vi "Format CSV.vi"(8 "error in (no error)":errorcluster, 9 "delimiter":string=",", 10 "CSV File Input":path, 11 "Original CSV Format":enum16{"Format A", "Format B"}(ring)) -> (0 "error out":errorcluster, 1 "Parcel Length":i32[](array[numeric]), 2 "All Terminal Data":T1(array[cluster]))   [LabVIEW 2017] (continued)
"36:44.6", "36:44.6", "36:44.6", "36:44.7", "36:44.7", "36:44.7", "36:44.8", "36:44.8", "36:44.8", "36:44.9", "36:44.9", "36:44.9", "36:45.0", "36:45.0", "36:45.0", "36:45.1", "36:45.1", "36:45.1", "36:45.2", "36:45.2", "36:45.2", "36:45.3", "36:45.3", "36:45.3", "36:45.4", "36:45.4", "36:45.4", "36:45.5", "36:45.5", "36:45.5", "36:45.6", "36:45.6", "36:45.6", "36:45.7", "36:45.7", "36:45.7", "36:45.8", "36:45.8", "36:45.8", "36:45.9", "36:45.9", "36:45.9", "36:46.0", "36:46.0", "36:46.0", "36:46.1", "36:46.1", "36:46.1", "36:46.2", "36:46.2", "36:46.2", "36:46.3", "36:46.3", "36:46.3", "36:46.4", "36:46.4", "36:46.4", "36:46.5", "36:46.5", "36:46.5", "36:46.6", "36:46.6", "36:46.6", "36:46.7", "36:46.7", "36:46.7", "36:46.8", "36:46.8", "36:46.8", "36:46.9", "36:46.9", "36:46.9", "36:47.0", "36:47.0", "36:47.0", "36:47.1", "36:47.1", "36:47.1", "36:47.2", "36:47.2", "36:47.2", "36:47.3", "36:47.3", "36:47.3", "36:47.4", "36:47.4", "36:47.4", "36:47.5", "36:47.5", "36:47.5", "36:47.6", "36:47.6", "36:47.6", "36:47.7", "36:47.7", "36:47.7", "36:47.8", "36:47.8", "36:47.8", "36:47.9", "36:47.9", "36:47.9", "36:48.0", "36:48.0", "36:48.0", "36:48.1", "36:48.1", "36:48.1", "36:48.2", "36:48.2", "36:48.2", "36:48.3", "36:48.3", "36:48.3", "36:48.4", "36:48.4", "36:48.4", "36:48.5", "36:48.5", "36:48.5", "36:48.6", "36:48.6", "36:48.6", "36:48.7", "36:48.7", "36:48.7", "36:48.8", "36:48.8", "36:48.8", "36:48.9", "36:48.9", "36:48.9", "36:49.0", "36:49.0", "36:49.0", "36:49.1", "36:49.1", "36:49.1", "36:49.2", "36:49.2", "36:49.2", "36:49.3", "36:49.3", "36:49.3", "36:49.4", "36:49.4", "36:49.4", "36:49.5", "36:49.5", "36:49.5", "36:49.6", "36:49.6", "36:49.6", "36:49.7", "36:49.7", "36:49.7", "36:49.8", "36:49.8", "36:49.8", "36:49.9", "36:49.9", "36:49.9", "36:50.0", "36:50.0", "36:50.0", "36:50.1", "36:50.1", "36:50.1", "36:50.2", "36:50.2", "36:50.2", "36:50.3", "36:50.3", "36:50.3", "36:50.4", "36:50.4", "36:50.4", "36:50.5", "36:50.5", "36:50.5", "36:50.6", "36:50.6", "36:50.6", "36:50.7", "36:50.7", "36:50.7", "36:50.8", "36:50.8", "36:50.8", "36:50.9", "36:50.9", "36:50.9", "36:51.0", "36:51.0", "36:51.0", "36:51.1", "36:51.1", "36:51.1", "36:51.2", "36:51.2", "36:51.2", "36:51.3", "36:51.3", "36:51.3", "36:51.4", "36:51.4", "36:51.4", "36:51.5", "36:51.5", "36:51.5", "36:51.6", "36:51.6", "36:51.6", "36:51.7", "36:51.7", "36:51.7", "36:51.8", "36:51.8", "36:51.8", "36:51.9", "36:51.9", "36:51.9", "36:52.0", "36:52.0", "36:52.0", "36:52.1", "36:52.1", "36:52.1", "36:52.2", "36:52.2", "36:52.2", "36:52.3", "36:52.3", "36:52.3", "36:52.4", "36:52.4", "36:52.4", "36:52.5", "36:52.5", "36:52.5", "36:52.6", "36:52.6", "36:52.6", "36:52.7", "36:52.7", "36:52.7", "36:52.8", "36:52.8", "36:52.8", "36:52.9", "36:52.9", "36:52.9", "36:53.0", "36:53.0", "36:53.0", "36:53.1", "36:53.1", "36:53.1", "36:53.2", "36:53.2", "36:53.2", "36:53.3", "36:53.3", "36:53.3", "36:53.4", "36:53.4", "36:53.4", "36:53.5", "36:53.5", "36:53.5", "36:53.6", "36:53.6", "36:53.6", "36:53.7", "36:53.7", "36:53.7", "36:53.8", "36:53.8", "36:53.8", "36:53.9", "36:53.9", "36:53.9", "36:54.0", "36:54.0", "36:54.0", "36:54.1", "36:54.1", "36:54.1", "36:54.2", "36:54.2", "36:54.2", "36:54.3", "36:54.3", "36:54.3", "36:54.4", "36:54.4", "36:54.4", "36:54.5", "36:54.5", "36:54.5", "36:54.6", "36:54.6", "36:54.6", "36:54.7", "36:54.7", "36:54.7", "36:54.8", "36:54.8", "36:54.8", "36:54.9", "36:54.9", "36:54.9", "36:55.0", "36:55.0", "36:55.0", "36:55.1", "36:55.1", "36:55.1", "36:55.2", "36:55.2", "36:55.2", "36:55.3", "36:55.3", "36:55.3", "36:55.4", "36:55.4", "36:55.4", "36:55.5", "36:55.5", "36:55.5", "36:55.6", "36:55.6", "36:55.6", "36:55.7", "36:55.7", "36:55.7", "36:55.8", "36:55.8", "36:55.8", "36:55.9", "36:55.9", "36:55.9", "36:56.0", "36:56.0", "36:56.0", "36:56.1", "36:56.1", "36:56.1", "36:56.2", "36:56.2", "36:56.2", "36:56.3", "36:56.3", "36:56.3", "36:56.4", "36:56.4", "36:56.4", "36:56.5", "36:56.5", "36:56.5", "36:56.6", "36:56.6", "36:56.6", "36:56.7", "36:56.7", "36:56.7", "36:56.8", "36:56.8", "36:56.8", "36:56.9", "36:56.9", "36:56.9", "36:57.0", "36:57.0", "36:57.0", "36:57.1", "36:57.1", "36:57.1", "36:57.2", "36:57.2", "36:57.2", "36:57.3", "36:57.3", "36:57.3", "36:57.4", "36:57.4", "36:57.4", "36:57.5", "36:57.5", "36:57.5", "36:57.6", "36:57.6", "36:57.6", "36:57.7", "36:57.7", "36:57.7", "36:57.8", "36:57.8", "36:57.8", "36:57.9", "36:57.9", "36:57.9", "36:58.0", "36:58.0", "36:58.0", "36:58.1", "36:58.1", "36:58.1", "36:58.2", "36:58.2", "36:58.2", "36:58.3", "36:58.3", "36:58.3", "36:58.4", "36:58.4", "36:58.4", "36:58.5", "36:58.5", "36:58.5", "36:58.6", "36:58.6", "36:58.6", "36:58.7", "36:58.7", "36:58.7", "36:58.8", "36:58.8", "36:58.8", "36:58.9", "36:58.9", "36:58.9", "36:59.0", "36:59.0", "36:59.0", "36:59.1", "36:59.1", "36:59.1", "36:59.2", "36:59.2", "36:59.2", "36:59.3", "36:59.3", "36:59.3", "36:59.4", "36:59.4", "36:59.4", "36:59.5", "36:59.5", "36:59.5", "36:59.6", "36:59.6", "36:59.6", "36:59.7", "36:59.7", "36:59.7", "36:59.8", "36:59.8", "36:59.8", "36:59.9", "36:59.9", "36:59.9", "37:00.0", "37:00.0", "37:00.0", "37:00.1", "37:00.1", "37:00.1", "37:00.2", "37:00.2", "37:00.2", "37:00.3", "37:00.3", "37:00.3", "37:00.4", "37:00.4", "37:00.4", "37:00.5", "37:00.5", "37:00.5", "37:00.6", "37:00.6", "37:00.6", "37:00.7", "37:00.7", "37:00.7", "37:00.8", "37:00.8", "37:00.8", "37:00.9", "37:00.9", "37:00.9", "37:01.0", "37:01.0", "37:01.0", "37:01.1", "37:01.1", "37:01.1", "37:01.2", "37:01.2", "37:01.2", "37:01.3", "37:01.3", "37:01.3", "37:01.4", "37:01.4", "37:01.4", "37:01.5", "37:01.5", "37:01.5", "37:01.6", "37:01.6", "37:01.6", "37:01.7", "37:01.7", "37:01.7", "37:01.8", "37:01.8", "37:01.8", "37:01.9", "37:01.9", "37:01.9", "37:02.0", "37:02.0", "37:02.0", "37:02.1", "37:02.1", "37:02.1", "37:02.2", "37:02.2", "37:02.2", "37:02.3", "37:02.3", "37:02.3", "37:02.4", "37:02.4", "37:02.4", "37:02.5", "37:02.5", "37:02.5", "37:02.6", "37:02.6", "37:02.6", "37:02.7", "37:02.7", "37:02.7", "37:02.8", "37:02.8", "37:02.8", "37:02.9", "37:02.9", "37:02.9", "37:03.0", "37:03.0", "37:03.0", "37:03.1", "37:03.1", "37:03.1", "37:03.2", "37:03.2", "37:03.2", "37:03.3", "37:03.3", "37:03.3", "37:03.4", "37:03.4", "37:03.4", "37:03.5", "37:03.5", "37:03.5", "37:03.6", "37:03.6", "37:03.6", "37:03.7", "37:03.7", "37:03.7", "37:03.8", "37:03.8", "37:03.8", "37:03.9", "37:03.9", "37:03.9", "37:04.0", "37:04.0", "37:04.0", "37:04.1", "37:04.1", "37:04.1", "37:04.2", "37:04.2", "37:04.2", "37:04.3", "37:04.3", "37:04.3", "37:04.4", "37:04.4", "37:04.4", "37:04.5", "37:04.5", "37:04.5", "37:04.6", "37:04.6", "37:04.6", "37:04.7", "37:04.7", "37:04.7", "37:04.8", "37:04.8", "37:04.8", "37:04.9", "37:04.9", "37:04.9", "37:05.0", "37:05.0", "37:05.0", "37:05.1", "37:05.1", "37:05.1", "37:05.2", "37:05.2", "37:05.2", "37:05.3", "37:05.3", "37:05.3", "37:05.4", "37:05.4", "37:05.4", "37:05.5", "37:05.5", "37:05.5", "37:05.6", "37:05.6", "37:05.6", "37:05.7", "37:05.7", "37:05.7", "37:05.8", "37:05.8", "37:05.8", "37:05.9", "37:05.9", "37:05.9", "37:06.0", "37:06.0", "37:06.0", "37:06.1", "37:06.1", "37:06.1", "37:06.2", "37:06.2", "37:06.2", "37:06.3", "37:06.3", "37:06.3", "37:06.4", "37:06.4", "37:06.4", "37:06.5", "37:06.5", "37:06.5", "37:06.6", "37:06.6", "37:06.6", "37:06.7", "37:06.7", "37:06.7", "37:06.8", "37:06.8", "37:06.8", "37:06.9", "37:06.9", "37:06.9", "37:07.0", "37:07.0", "37:07.0", "37:07.1", "37:07.1", "37:07.1", "37:07.2", "37:07.2", "37:07.2", "37:07.3", "37:07.3", "37:07.3", "37:07.4", "37:07.4", "37:07.4", "37:07.5", "37:07.5", "37:07.5", "37:07.6", "37:07.6", "37:07.6", "37:07.7", "37:07.7", "37:07.7", "37:07.8", "37:07.8", "37:07.8", "37:07.9", "37:07.9", "37:07.9", "37:08.0", "37:08.0", "37:08.0", "37:08.1", "37:08.1", "37:08.1", "37:08.2", "37:08.2", "37:08.2", "37:08.3", "37:08.3", "37:08.3", "37:08.4", "37:08.4", "37:08.4", "37:08.5", "37:08.5", "37:08.5", "37:08.6", "37:08.6", "37:08.6", "37:08.7", "37:08.7", "37:08.7", "37:08.8", "37:08.8", "37:08.8", "37:08.9", "37:08.9", "37:08.9", "37:09.0", "37:09.0", "37:09.0", "37:09.1", "37:09.1", "37:09.1", "37:09.2", "37:09.2", "37:09.2", "37:09.3", "37:09.3", "37:09.3", "37:09.4", "37:09.4", "37:09.4", "37:09.5", "37:09.5", "37:09.5", "37:09.6", "37:09.6", "37:09.6", "37:09.7", "37:09.7", "37:09.7", "37:09.8", "37:09.8", "37:09.8", "37:09.9", "37:09.9", "37:09.9", "37:10.0", "37:10.0", "37:10.0", "37:10.1", "37:10.1", "37:10.1", "37:10.2", "37:10.2", "37:10.2", "37:10.3", "37:10.3", "37:10.3", "37:10.4", "37:10.4", "37:10.4", "37:10.5", "37:10.5", "37:10.5", "37:10.6", "37:10.6", "37:10.6", "37:10.7", "37:10.7", "37:10.7", "37:10.8", "37:10.8", "37:10.8", "37:10.9", "37:10.9", "37:10.9", "37:11.0", "37:11.0", "37:11.0", "37:11.1", "37:11.1", "37:11.1", "37:11.2", "37:11.2", "37:11.2", "37:11.3", "37:11.3", "37:11.3", "37:11.4", "37:11.4", "37:11.4", "37:11.5", "37:11.5", "37:11.5", "37:11.6", "37:11.6", "37:11.6", "37:11.7", "37:11.7", "37:11.7", "37:11.8", "37:11.8", "37:11.8", "37:11.9", "37:11.9", "37:11.9", "37:12.0", "37:12.0", "37:12.0", "37:12.1", "37:12.1", "37:12.1", "37:12.2", "37:12.2", "37:12.2", "37:12.3", "37:12.3", "37:12.3", "37:12.4", "37:12.4", "37:12.4", "37:12.5", "37:12.5", "37:12.5", "37:12.6", "37:12.6", "37:12.6", "37:12.7", "37:12.7", "37:12.7", "37:12.8", "37:12.8", "37:12.8", "37:12.9", "37:12.9", "37:12.9", "37:13.0", "37:13.0", "37:13.0", "37:13.1", "37:13.1", "37:13.1", "37:13.2", "37:13.2", "37:13.2", "37:13.3", "37:13.3", "37:13.3", "37:13.4", "37:13.4", "37:13.4", "37:13.5", "37:13.5", "37:13.5", "37:13.6", "37:13.6", "37:13.6", "37:13.7", "37:13.7", "37:13.7", "37:13.8", "37:13.8", "37:13.8", "37:13.9", "37:13.9", "37:13.9", "37:14.0", "37:14.0", "37:14.0", "37:14.1", "37:14.1", "37:14.1", "37:14.2", "37:14.2", "37:14.2", "37:14.3", "37:14.3", "37:14.3", "37:14.4", "37:14.4", "37:14.4", "37:14.5", "37:14.5", "37:14.5", "37:14.6", "37:14.6", "37:14.6", "37:14.7", "37:14.7", "37:14.7", "37:14.8", "37:14.8", "37:14.8", "37:14.9", "37:14.9", "37:14.9", "37:15.0", "37:15.0", "37:15.0", "37:15.1", "37:15.1", "37:15.1", "37:15.2", "37:15.2", "37:15.2", "37:15.3", "37:15.3", "37:15.3", "37:15.4", "37:15.4", "37:15.4", "37:15.5", "37:15.5", "37:15.5", "37:15.6", "37:15.6", "37:15.6", "37:15.7", "37:15.7", "37:15.7", "37:15.8", "37:15.8", "37:15.8", "37:15.9", "37:15.9", "37:15.9", "37:16.0", "37:16.0", "37:16.0", "37:16.1", "37:16.1", "37:16.1", "37:16.2", "37:16.2", "37:16.2", "37:16.3", "37:16.3", "37:16.3", "37:16.4", "37:16.4", "37:16.4", "37:16.5", "37:16.5", "37:16.5", "37:16.6", "37:16.6", "37:16.6", "37:16.7", "37:16.7", "37:16.7", "37:16.8", "37:16.8", "37:16.8", "37:16.9", "37:16.9", "37:16.9", "37:17.0", "37:17.0", "37:17.0", "37:17.1", "37:17.1", "37:17.1", "37:17.2", "37:17.2", "37:17.2", "37:17.3", "37:17.3", "37:17.3", "37:17.4", "37:17.4", "37:17.4", "37:17.5", "37:17.5", "37:17.5", "37:17.6", "37:17.6", "37:17.6", "37:17.7", "37:17.7", "37:17.7", "37:17.8", "37:17.8", "37:17.8", "37:17.9", "37:17.9", "37:17.9", "37:18.0", "37:18.0", "37:18.0", "37:18.1", "37:18.1", "37:18.1", "37:18.2", "37:18.2", "37:18.2", "37:18.3", "37:18.3", "37:18.3", "37:18.4", "37:18.4", "37:18.4", "37:18.5", "37:18.5", "37:18.5", "37:18.6", "37:18.6", "37:18.6", "37:18.7", "37:18.7", "37:18.7", "37:18.8", "37:18.8", "37:18.8", "37:18.9", "37:18.9", "37:18.9", "37:19.0", "37:19.0", "37:19.0", "37:19.1", "37:19.1", "37:19.1", "37:19.2", "37:19.2", "37:19.2", "37:19.3", "37:19.3", "37:19.3", "37:19.4", "37:19.4", "37:19.4", "37:19.5", "37:19.5", "37:19.5", "37:19.6", "37:19.6", "37:19.6", "37:19.7", "37:19.7", "37:19.7", "37:19.8", "37:19.8", "37:19.8", "37:19.9", "37:19.9", "37:19.9", "37:20.0", "37:20.0", "37:20.0", "37:20.1", "37:20.1", "37:20.1", "37:20.2", "37:20.2", "37:20.2", "37:20.3", "37:20.3", "37:20.3", "37:20.4", "37:20.4", "37:20.4", "37:20.5", "37:20.5", "37:20.5", "37:20.6", "37:20.6", "37:20.6", "37:20.7", "37:20.7", "37:20.7", "37:20.8", "37:20.8", "37:20.8", "37:20.9", "37:20.9", "37:20.9", "37:21.0", "37:21.0", "37:21.0", "37:21.1", "37:21.1", "37:21.1", "37:21.2", "37:21.2", "37:21.2", "37:21.3", "37:21.3", "37:21.3", "37:21.4", "37:21.4", "37:21.4", "37:21.5", "37:21.5", "37:21.5", "37:21.6", "37:21.6", "37:21.6", "37:21.7", "37:21.7", "37:21.7", "37:21.8", "37:21.8", "37:21.8", "37:21.9", "37:21.9", "37:21.9", "37:22.0", "37:22.0", "37:22.0", "37:22.1", "37:22.1", "37:22.1", "37:22.2", "37:22.2", "37:22.2", "37:22.3", "37:22.3", "37:22.3", "37:22.4", "37:22.4", "37:22.4", "37:22.5", "37:22.5", "37:22.5", "37:22.6", "37:22.6", "37:22.6", "37:22.7", "37:22.7", "37:22.7", "37:22.8", "37:22.8", "37:22.8", "37:22.9", "37:22.9", "37:22.9", "37:23.0", "37:23.0", "37:23.0", "37:23.1", "37:23.1", "37:23.1", "37:23.2", "37:23.2", "37:23.2", "37:23.3", "37:23.3", "37:23.3", "37:23.4", "37:23.4", "37:23.4", "37:23.5", "37:23.5", "37:23.5", "37:23.6", "37:23.6", "37:23.6", "37:23.7", "37:23.7", "37:23.7", "37:23.8", "37:23.8", "37:23.8", "37:23.9", "37:23.9", "37:23.9", "37:24.0", "37:24.0", "37:24.0", "37:24.1", "37:24.1", "37:24.1", "37:24.2", "37:24.2", "37:24.2", "37:24.3", "37:24.3", "37:24.3", "37:24.4", "37:24.4", "37:24.4", "37:24.5", "37:24.5", "37:24.5", "37:24.6", "37:24.6", "37:24.6", "37:24.7", "37:24.7", "37:24.7", "37:24.8", "37:24.8", "37:24.8", "37:24.9", "37:24.9", "37:24.9", "37:25.0", "37:25.0", "37:25.0", "37:25.1", "37:25.1", "37:25.1", "37:25.2", "37:25.2", "37:25.2", "37:25.3", "37:25.3", "37:25.3", "37:25.4", "37:25.4", "37:25.4", "37:25.5", "37:25.5", "37:25.5", "37:25.6", "37:25.6", "37:25.6", "37:25.7", "37:25.7", "37:25.7", "37:25.8", "37:25.8", "37:25.8", "37:25.9", "37:25.9", "37:25.9", "37:26.0", "37:26.0", "37:26.0", "37:26.1", "37:26.1", "37:26.1", "37:26.2", "37:26.2", "37:26.2", "37:26.3", "37:26.3", "37:26.3", "37:26.4", "37:26.4", "37:26.4", "37:26.5", "37:26.5", "37:26.5", "37:26.6", "37:26.6", "37:26.6", "37:26.7", "37:26.7", "37:26.7", "37:26.8", "37:26.8", "37:26.8", "37:26.9", "37:26.9", "37:26.9", "37:27.0", "37:27.0", "37:27.0", "37:27.1", "37:27.1", "37:27.1", "37:27.2", "37:27.2", "37:27.2", "37:27.3", "37:27.3", "37:27.3", "37:27.4", "37:27.4", "37:27.4", "37:27.5", "37:27.5", "37:27.5", "37:27.6", "37:27.6", "37:27.6", "37:27.7", "37:27.7", "37:27.7", "37:27.8", "37:27.8", "37:27.8", "37:27.9", "37:27.9", "37:27.9", "37:28.0", "37:28.0", "37:28.0", "37:28.1", "37:28.1", "37:28.1", "37:28.2", "37:28.2", "37:28.2", "37:28.3", "37:28.3", "37:28.3", "37:28.4", "37:28.4", "37:28.4", "37:28.5", "37:28.5", "37:28.5", "37:28.6", "37:28.6", "37:28.6", "37:28.7", "37:28.7", "37:28.7", "37:28.8", "37:28.8", "37:28.8", "37:28.9", "37:28.9", "37:28.9", "37:29.0", "37:29.0", "37:29.0", "37:29.1", "37:29.1", "37:29.1", "37:29.2", "37:29.2", "37:29.2", "37:29.3", "37:29.3", "37:29.3", "37:29.4", "37:29.4", "37:29.4", "37:29.5", "37:29.5", "37:29.5", "37:29.6", "37:29.6", "37:29.6", "37:29.7", "37:29.7", "37:29.7", "37:29.8", "37:29.8", "37:29.8", "37:29.9", "37:29.9", "37:29.9", "37:30.0", "37:30.0", "37:30.0", "37:30.1", "37:30.1", "37:30.1", "37:30.2", "37:30.2", "37:30.2", "37:30.3", "37:30.3", "37:30.3", "37:30.4", "37:30.4", "37:30.4", "37:30.5", "37:30.5", "37:30.5", "37:30.6", "37:30.6", "37:30.6", "37:30.7", "37:30.7", "37:30.7", "37:30.8", "37:30.8", "37:30.8", "37:30.9", "37:30.9", "37:30.9", "37:31.0", "37:31.0", "37:31.0", "37:31.1", "37:31.1", "37:31.1", "37:31.2", "37:31.2", "37:31.2", "37:31.3", "37:31.3", "37:31.3", "37:31.4", "37:31.4", "37:31.4", "37:31.5", "37:31.5", "37:31.5", "37:31.6", "37:31.6", "37:31.6", "37:31.7", "37:31.7", "37:31.7", "37:31.8", "37:31.8", "37:31.8", "37:31.9", "37:31.9", "37:31.9", "37:32.0", "37:32.0", "37:32.0", "37:32.1", "37:32.1", "37:32.1", "37:32.2", "37:32.2", "37:32.2", "37:32.3", "37:32.3", "37:32.3", "37:32.4", "37:32.4", "37:32.4", "37:32.5", "37:32.5", "37:32.5", "37:32.6", "37:32.6", "37:32.6", "37:32.7", "37:32.7", "37:32.7", "37:32.8", "37:32.8", "37:32.8", "37:32.9", "37:32.9", "37:32.9", "37:33.0", "37:33.0", "37:33.0", "37:33.1", "37:33.1", "37:33.1", "37:33.2", "37:33.2", "37:33.2", "37:33.3", "37:33.3", "37:33.3", "37:33.4", "37:33.4", "37:33.4", "37:33.5", "37:33.5", "37:33.5", "37:33.6", "37:33.6", "37:33.6", "37:33.7", "37:33.7", "37:33.7", "37:33.8", "37:33.8", "37:33.8", "37:33.9", "37:33.9", "37:33.9", "37:34.0", "37:34.0", "37:34.0", "37:34.1", "37:34.1", "37:34.1", "37:34.2", "37:34.2", "37:34.2", "37:34.3", "37:34.3", "37:34.3", "37:34.4", "37:34.4", "37:34.4", "37:34.5", "37:34.5", "37:34.5", "37:34.6", "37:34.6", "37:34.6", "37:34.7", "37:34.7", "37:34.7", "37:34.8", "37:34.8", "37:34.8", "37:34.9", "37:34.9", "37:34.9", "37:35.0", "37:35.0", "37:35.0", "37:35.1", "37:35.1", "37:35.1", "37:35.2", "37:35.2", "37:35.2", "37:35.3", "37:35.3", "37:35.3", "37:35.4", "37:35.4", "37:35.4", "37:35.5", "37:35.5", "37:35.5", "37:35.6", "37:35.6", "37:35.6", "37:35.7", "37:35.7", "37:35.7", "37:35.8", "37:35.8", "37:35.8", "37:35.9", "37:35.9", "37:35.9", "37:36.0", "37:36.0", "37:36.0", "37:36.1", "37:36.1", "37:36.1", "37:36.2", "37:36.2", "37:36.2", "37:36.3", "37:36.3", "37:36.3", "37:36.4", "37:36.4", "37:36.4", "37:36.5", "37:36.5", "37:36.5", "37:36.6", "37:36.6", "37:36.6", "37:36.7", "37:36.7", "37:36.7", "37:36.8", "37:36.8", "37:36.8", "37:36.9", "37:36.9", "37:36.9", "37:37.0", "37:37.0", "37:37.0", "37:37.1", "37:37.1", "37:37.1", "37:37.2", "37:37.2", "37:37.2", "37:37.3", "37:37.3", "37:37.3", "37:37.4", "37:37.4", "37:37.4", "37:37.5", "37:37.5", "37:37.5", "37:37.6", "37:37.6", "37:37.6", "37:37.7", "37:37.7", "37:37.7", "37:37.8", "37:37.8", "37:37.8", "37:37.9", "37:37.9", "37:37.9", "37:38.0", "37:38.0", "37:38.0", "37:38.1", "37:38.1", "37:38.1", "37:38.2", "37:38.2", "37:38.2", "37:38.3", "37:38.3", "37:38.3", "37:38.4", "37:38.4", "37:38.4", "37:38.5", "37:38.5", "37:38.5", "37:38.6", "37:38.6", "37:38.6", "37:38.7", "37:38.7", "37:38.7", "37:38.8", "37:38.8", "37:38.8", "37:38.9", "37:38.9", "37:38.9", "37:39.0", "37:39.0", "37:39.0", "37:39.1", "37:39.1", "37:39.1", "37:39.2", "37:39.2", "37:39.2", "37:39.3", "37:39.3", "37:39.3", "37:39.4", "37:39.4", "37:39.4", "37:39.5", "37:39.5", "37:39.5", "37:39.6", "37:39.6", "37:39.6", "37:39.7", "37:39.7", "37:39.7", "37:39.8", "37:39.8", "37:39.8", "37:39.9", "37:39.9", "37:39.9", "37:40.0", "37:40.0", "37:40.0", "37:40.1", "37:40.1", "37:40.1", "37:40.2", "37:40.2", "37:40.2", "37:40.3", "37:40.3", "37:40.3", "37:40.4", "37:40.4", "37:40.4", "37:40.5", "37:40.5", "37:40.5", "37:40.6", "37:40.6", "37:40.6", "37:40.7", "37:40.7", "37:40.7", "37:40.8", "37:40.8", "37:40.8", "37:40.9", "37:40.9", "37:40.9", "37:41.0", "37:41.0", "37:41.0", "37:41.1", "37:41.1", "37:41.1", "37:41.2", "37:41.2", "37:41.2", "37:41.3", "37:41.3", "37:41.3", "37:41.4", "37:41.4", "37:41.4", "37:41.5", "37:41.5", "37:41.5", "37:41.6", "37:41.6", "37:41.6", "37:41.7", "37:41.7", "37:41.7", "37:41.8", "37:41.8", "37:41.8", "37:41.9", "37:41.9", "37:41.9", "37:42.0", "37:42.0", "37:42.0", "37:42.1", "37:42.1", "37:42.1", "37:42.2", "37:42.2", "37:42.2", "37:42.3", "37:42.3", "37:42.3", "37:42.4", "37:42.4", "37:42.4", "37:42.5", "37:42.5", "37:42.5", "37:42.6", "37:42.6", "37:42.6", "37:42.7", "37:42.7", "37:42.7", "37:42.8", "37:42.8", "37:42.8", "37:42.9", "37:42.9", "37:42.9", "37:43.0", "37:43.0", "37:43.0", "37:43.1", "37:43.1", "37:43.1", "37:43.2", "37:43.2", "37:43.2", "37:43.3", "37:43.3", "37:43.3", "37:43.4", "37:43.4", "37:43.4", "37:43.5", "37:43.5", "37:43.5", "37:43.6", "37:43.6", "37:43.6", "37:43.7", "37:43.7", "37:43.7", "37:43.8", "37:43.8", "37:43.8", "37:43.9", "37:43.9", "37:43.9", "37:44.0", "37:44.0", "37:44.0", "37:44.1", "37:44.1", "37:44.1", "37:44.2", "37:44.2", "37:44.2", "37:44.3", "37:44.3", "37:44.3", "37:44.4", "37:44.4", "37:44.4", "37:44.5", "37:44.5", "37:44.5", "37:44.6", "37:44.6", "37:44.6", "37:44.7", "37:44.7", "37:44.7", "37:44.8", "37:44.8", "37:44.8", "37:44.9", "37:44.9", "37:44.9", "37:45.0", "37:45.0", "37:45.0", "37:45.1", "37:45.1", "37:45.1", "37:45.2", "37:45.2", "37:45.2", "37:45.3", "37:45.3", "37:45.3", "37:45.4", "37:45.4", "37:45.4", "37:45.5", "37:45.5", "37:45.5", "37:45.6", "37:45.6", "37:45.6", "37:45.7", "37:45.7", "37:45.7", "37:45.8", "37:45.8", "37:45.8", "37:45.9", "37:45.9", "37:45.9", "37:46.0", "37:46.0", "37:46.0", "37:46.1", "37:46.1", "37:46.1", "37:46.2", "37:46.2", "37:46.2", "37:46.3", "37:46.3", "37:46.3", "37:46.4", "37:46.4", "37:46.4", "37:46.5", "37:46.5", "37:46.5", "37:46.6", "37:46.6", "37:46.6", "37:46.7", "37:46.7", "37:46.7", "37:46.8", "37:46.8", "37:46.8", "37:46.9", "37:46.9", "37:46.9", "37:47.0", "37:47.0", "37:47.0", "37:47.1", "37:47.1", "37:47.1", "37:47.2", "37:47.2", "37:47.2", "37:47.3", "37:47.3", "37:47.3", "37:47.4", "37:47.4", "37:47.4", "37:47.5", "37:47.5", "37:47.5", "37:47.6", "37:47.6", "37:47.6", "37:47.7", "37:47.7", "37:47.7", "37:47.8", "37:47.8", "37:47.8", "37:47.9", "37:47.9", "37:47.9", "37:48.0", "37:48.0", "37:48.0", "37:48.1", "37:48.1", "37:48.1", "37:48.2", "37:48.2", "37:48.2", "37:48.3", "37:48.3", "37:48.3", "37:48.4", "37:48.4", "37:48.4", "37:48.5", "37:48.5", "37:48.5", "37:48.6", "37:48.6", "37:48.6", "37:48.7", "37:48.7", "37:48.7", "37:48.8", "37:48.8", "37:48.8", "37:48.9", "37:48.9", "37:48.9", "37:49.0", "37:49.0", "37:49.0", "37:49.1", "37:49.1", "37:49.1", "37:49.2", "37:49.2", "37:49.2", "37:49.3", "37:49.3", "37:49.3", "37:49.4", "37:49.4", "37:49.4", "37:49.5", "37:49.5", "37:49.5", "37:49.6", "37:49.6", "37:49.6", "37:49.7", "37:49.7", "37:49.7", "37:49.8", "37:49.8", "37:49.8", "37:49.9", "37:49.9", "37:49.9", "37:50.0", "37:50.0", "37:50.0", "37:50.1", "37:50.1", "37:50.1", "37:50.2", "37:50.2", "37:50.2", "37:50.3", "37:50.3", "37:50.3", "37:50.4", "37:50.4", "37:50.4", "37:50.5", "37:50.5", "37:50.5", "37:50.6", "37:50.6", "37:50.6", "37:50.7", "37:50.7", "37:50.7", "37:50.8", "37:50.8", "37:50.8", "37:50.9", "37:50.9", "37:50.9", "37:51.0", "37:51.0", "37:51.0", "37:51.1", "37:51.1", "37:51.1", "37:51.2", "37:51.2", "37:51.2", "37:51.3", "37:51.3", "37:51.3", "37:51.4", "37:51.4", "37:51.4", "37:51.5", "37:51.5", "37:51.5", "37:51.6", "37:51.6", "37:51.6", "37:51.7", "37:51.7", "37:51.7", "37:51.8", "37:51.8", "37:51.8", "37:51.9", "37:51.9", "37:51.9", "37:52.0", "37:52.0", "37:52.0", "37:52.1", "37:52.1", "37:52.1", "37:52.2", "37:52.2", "37:52.2", "37:52.3", "37:52.3", "37:52.3", "37:52.4", "37:52.4", "37:52.4", "37:52.5", "37:52.5", "37:52.5", "37:52.6", "37:52.6", "37:52.6", "37:52.7", "37:52.7", "37:52.7", "37:52.8", "37:52.8", "37:52.8", "37:52.9", "37:52.9", "37:52.9", "37:53.0", "37:53.0", "37:53.0", "37:53.1", "37:53.1", "37:53.1", "37:53.2", "37:53.2", "37:53.2", "37:53.3", "37:53.3", "37:53.3", "37:53.4", "37:53.4", "37:53.4", "37:53.5", "37:53.5", "37:53.5", "37:53.6", "37:53.6", "37:53.6", "37:53.7", "37:53.7", "37:53.7", "37:53.8", "37:53.8", "37:53.8", "37:53.9", "37:53.9", "37:53.9", "37:54.0", "37:54.0", "37:54.0", "37:54.1", "37:54.1", "37:54.1", "37:54.2", "37:54.2", "37:54.2", "37:54.3", "37:54.3", "37:54.3", "37:54.4", "37:54.4", "37:54.4", "37:54.5", "37:54.5", "37:54.5", "37:54.6", "37:54.6", "37:54.6", "37:54.7", "37:54.7", "37:54.7", "37:54.8", "37:54.8", "37:54.8", "37:54.9", "37:54.9", "37:54.9", "37:55.0", "37:55.0", "37:55.0", "37:55.1", "37:55.1", "37:55.1", "37:55.2", "37:55.2", "37:55.2", "37:55.3", "37:55.3", "37:55.3", "37:55.4", "37:55.4", "37:55.4", "37:55.5", "37:55.5", "37:55.5", "37:55.6", "37:55.6", "37:55.6", "37:55.7", "37:55.7", "37:55.7", "37:55.8", "37:55.8", "37:55.8", "37:55.9", "37:55.9", "37:55.9", "37:56.0", "37:56.0", "37:56.0", "37:56.1", "37:56.1", "37:56.1", "37:56.2", "37:56.2", "37:56.2", "37:56.3", "37:56.3", "37:56.3", "37:56.4", "37:56.4", "37:56.4", "37:56.5", "37:56.5", "37:56.5", "37:56.6", "37:56.6", "37:56.6", "37:56.7", "37:56.7", "37:56.7", "37:56.8", "37:56.8", "37:56.8", "37:56.9", "37:56.9", "37:56.9", "37:57.0", "37:57.0", "37:57.0", "37:57.1", "37:57.1", "37:57.1", "37:57.2", "37:57.2", "37:57.2", "37:57.3", "37:57.3", "37:57.3", "37:57.4", "37:57.4", "37:57.4", "37:57.5", "37:57.5", "37:57.5", "37:57.6", "37:57.6", "37:57.6", "37:57.7", "37:57.7", "37:57.7", "37:57.8", "37:57.8", "37:57.8", "37:57.9", "37:57.9", "37:57.9", "37:58.0", "37:58.0", "37:58.0", "37:58.1", "37:58.1", "37:58.1", "37:58.2", "37:58.2", "37:58.2", "37:58.3", "37:58.3", "37:58.3", "37:58.4", "37:58.4", "37:58.4", "37:58.5", "37:58.5", "37:58.5", "37:58.6", "37:58.6", "37:58.6", "37:58.7", "37:58.7", "37:58.7", "37:58.8", "37:58.8", "37:58.8", "37:58.9", "37:58.9", "37:58.9", "37:59.0", "37:59.0", "37:59.0", "37:59.1", "37:59.1", "37:59.1", "37:59.2", "37:59.2", "37:59.2", "37:59.3", "37:59.3", "37:59.3", "37:59.4", "37:59.4", "37:59.4", "37:59.5", "37:59.5", "37:59.5", "37:59.6", "37:59.6", "37:59.6", "37:59.7", "37:59.7", "37:59.7", "37:59.8", "37:59.8", "37:59.8", "37:59.9", "37:59.9", "37:59.9", "38:00.0", "38:00.0", "38:00.0", "38:00.1", "38:00.1", "38:00.1", "38:00.2", "38:00.2", "38:00.2", "38:00.3", "38:00.3", "38:00.3", "38:00.4", "38:00.4", "38:00.4", "38:00.5", "38:00.5", "38:00.5", "38:00.6", "38:00.6", "38:00.6", "38:00.7", "38:00.7", "38:00.7", "38:00.8", "38:00.8", "38:00.8", "38:00.9", "38:00.9", "38:00.9", "38:01.0", "38:01.0", "38:01.0", "38:01.1", "38:01.1", "38:01.1", "38:01.2", "38:01.2", "38:01.2", "38:01.3", "38:01.3", "38:01.3", "38:01.4", "38:01.4", "38:01.4", "38:01.5", "38:01.5", "38:01.5", "38:01.6", "38:01.6", "38:01.6", "38:01.7", "38:01.7", "38:01.7", "38:01.8", "38:01.8", "38:01.8", "38:01.9", "38:01.9", "38:01.9", "38:02.0", "38:02.0", "38:02.0", "38:02.1", "38:02.1", "38:02.1", "38:02.2", "38:02.2", "38:02.2", "38:02.3", "38:02.3", "38:02.3", "38:02.4", "38:02.4", "38:02.4", "38:02.5", "38:02.5", "38:02.5", "38:02.6", "38:02.6", "38:02.6", "38:02.7", "38:02.7", "38:02.7", "38:02.8", "38:02.8", "38:02.8", "38:02.9", "38:02.9", "38:02.9", "38:03.0", "38:03.0", "38:03.0", "38:03.1", "38:03.1", "38:03.1", "38:03.2", "38:03.2", "38:03.2", "38:03.3", "38:03.3", "38:03.3", "38:03.4", "38:03.4", "38:03.4", "38:03.5", "38:03.5", "38:03.5", "38:03.6", "38:03.6", "38:03.6", "38:03.7", "38:03.7", "38:03.7", "38:03.8", "38:03.8", "38:03.8", "38:03.9", "38:03.9", "38:03.9", "38:04.0", "38:04.0", "38:04.0", "38:04.1", "38:04.1", "38:04.1", "38:04.2", "38:04.2", "38:04.2", "38:04.3", "38:04.3", "38:04.3", "38:04.4", "38:04.4", "38:04.4", "38:04.5", "38:04.5", "38:04.5", "38:04.6", "38:04.6", "38:04.6", "38:04.7", "38:04.7", "38:04.7", "38:04.8", "38:04.8", "38:04.8", "38:04.9", "38:04.9", "38:04.9", "38:05.0", "38:05.0", "38:05.0", "38:05.1", "38:05.1", "38:05.1", "38:05.2", "38:05.2", "38:05.2", "38:05.3", "38:05.3", "38:05.3", "38:05.4", "38:05.4", "38:05.4", "38:05.5", "38:05.5", "38:05.5", "38:05.6", "38:05.6", "38:05.6", "38:05.7", "38:05.7", "38:05.7", "38:05.8", "38:05.8", "38:05.8", "38:05.9", "38:05.9", "38:05.9", "38:06.0", "38:06.0", "38:06.0", "38:06.1", "38:06.1", "38:06.1", "38:06.2", "38:06.2", "38:06.2", "38:06.3", "38:06.3", "38:06.3", "38:06.4", "38:06.4", "38:06.4", "38:06.5", "38:06.5", "38:06.5", "38:06.6", "38:06.6", "38:06.6", "38:06.7", "38:06.7", "38:06.7", "38:06.8", "38:06.8", "38:06.8", "38:06.9", "38:06.9", "38:06.9", "38:07.0", "38:07.0", "38:07.0", "38:07.1", "38:07.1", "38:07.1", "38:07.2", "38:07.2", "38:07.2", "38:07.3", "38:07.3", "38:07.3", "38:07.4", "38:07.4", "38:07.4", "38:07.5", "38:07.5", "38:07.5", "38:07.6", "38:07.6", "38:07.6", "38:07.7", "38:07.7", "38:07.7", "38:07.8", "38:07.8", "38:07.8", "38:07.9", "38:07.9", "38:07.9", "38:08.0", "38:08.0", "38:08.0", "38:08.1", "38:08.1", "38:08.1", "38:08.2", "38:08.2", "38:08.2", "38:08.3", "38:08.3", "38:08.3", "38:08.4", "38:08.4", "38:08.4", "38:08.5", "38:08.5", "38:08.5", "38:08.6", "38:08.6", "38:08.6", "38:08.7", "38:08.7", "38:08.7", "38:08.8", "38:08.8", "38:08.8", "38:08.9", "38:08.9", "38:08.9", "38:09.0", "38:09.0", "38:09.0", "38:09.1", "38:09.1", "38:09.1", "38:09.2", "38:09.2", "38:09.2", "38:09.3", "38:09.3", "38:09.3", "38:09.4", "38:09.4", "38:09.4", "38:09.5", "38:09.5", "38:09.5", "38:09.6", "38:09.6", "38:09.6", "38:09.7", "38:09.7", "38:09.7", "38:09.8", "38:09.8", "38:09.8", "38:09.9", "38:09.9", "38:09.9", "38:10.0", "38:10.0", "38:10.0", "38:10.1", "38:10.1", "38:10.1", "38:10.2", "38:10.2", "38:10.2", "38:10.3", "38:10.3", "38:10.3", "38:10.4", "38:10.4", "38:10.4", "38:10.5", "38:10.5", "38:10.5", "38:10.6", "38:10.6", "38:10.6", "38:10.7", "38:10.7", "38:10.7", "38:10.8", "38:10.8", "38:10.8", "38:10.9", "38:10.9", "38:10.9", "38:11.0", "38:11.0", "38:11.0", "38:11.1", "38:11.1", "38:11.1", "38:11.2", "38:11.2", "38:11.2", "38:11.3", "38:11.3", "38:11.3", "38:11.4", "38:11.4", "38:11.4", "38:11.5", "38:11.5", "38:11.5", "38:11.6", "38:11.6", "38:11.6", "38:11.7", "38:11.7", "38:11.7", "38:11.8", "38:11.8", "38:11.8", "38:11.9", "38:11.9", "38:11.9", "38:12.0", "38:12.0", "38:12.0", "38:12.1", "38:12.1", "38:12.1", "38:12.2", "38:12.2", "38:12.2", "38:12.3", "38:12.3", "38:12.3", "38:12.4", "38:12.4", "38:12.4", "38:12.5", "38:12.5", "38:12.5", "38:12.6", "38:12.6", "38:12.6", "38:12.7", "38:12.7", "38:12.7", "38:12.8", "38:12.8", "38:12.8", "38:12.9", "38:12.9", "38:12.9", "38:13.0", "38:13.0", "38:13.0", "38:13.1", "38:13.1", "38:13.1", "38:13.2", "38:13.2", "38:13.2", "38:13.3", "38:13.3", "38:13.3", "38:13.4", "38:13.4", "38:13.4", "38:13.5", "38:13.5", "38:13.5", "38:13.6", "38:13.6", "38:13.6", "38:13.7", "38:13.7", "38:13.7", "38:13.8", "38:13.8", "38:13.8", "38:13.9", "38:13.9", "38:13.9", "38:14.0", "38:14.0", "38:14.0", "38:14.1", "38:14.1", "38:14.1", "38:14.2", "38:14.2", "38:14.2", "38:14.3", "38:14.3", "38:14.3", "38:14.4", "38:14.4", "38:14.4", "38:14.5", "38:14.5", "38:14.5", "38:14.6", "38:14.6", "38:14.6", "38:14.7", "38:14.7", "38:14.7", "38:14.8", "38:14.8", "38:14.8", "38:14.9", "38:14.9", "38:14.9", "38:15.0", "38:15.0", "38:15.0", "38:15.1", "38:15.1", "38:15.1", "38:15.2", "38:15.2", "38:15.2", "38:15.3", "38:15.3", "38:15.3", "38:15.4", "38:15.4", "38:15.4", "38:15.5", "38:15.5", "38:15.5", "38:15.6", "38:15.6", "38:15.6", "38:15.7", "38:15.7", "38:15.7", "38:15.8", "38:15.8", "38:15.8", "38:15.9", "38:15.9", "38:15.9", "38:16.0", "38:16.0", "38:16.0", "38:16.1", "38:16.1", "38:16.1", "38:16.2", "38:16.2", "38:16.2", "38:16.3", "38:16.3", "38:16.3", "38:16.4", "38:16.4", "38:16.4", "38:16.5", "38:16.5", "38:16.5", "38:16.6", "38:16.6", "38:16.6", "38:16.7", "38:16.7", "38:16.7", "38:16.8", "38:16.8", "38:16.8", "38:16.9", "38:16.9", "38:16.9", "38:17.0", "38:17.0", "38:17.0", "38:17.1", "38:17.1", "38:17.1", "38:17.2", "38:17.2", "38:17.2", "38:17.3", "38:17.3", "38:17.3", "38:17.4", "38:17.4", "38:17.4", "38:17.5", "38:17.5", "38:17.5", "38:17.6", "38:17.6", "38:17.6", "38:17.7", "38:17.7", "38:17.7", "38:17.8", "38:17.8", "38:17.8", "38:17.9", "38:17.9", "38:17.9", "38:18.0", "38:18.0", "38:18.0", "38:18.1", "38:18.1", "38:18.1", "38:18.2", "38:18.2", "38:18.2", "38:18.3", "38:18.3", "38:18.3", "38:18.4", "38:18.4", "38:18.4", "38:18.5", "38:18.5", "38:18.5", "38:18.6", "38:18.6", "38:18.6", "38:18.7", "38:18.7", "38:18.7", "38:18.8", "38:18.8", "38:18.8", "38:18.9", "38:18.9", "38:18.9", "38:19.0", "38:19.0", "38:19.0", "38:19.1", "38:19.1", "38:19.1", "38:19.2", "38:19.2", "38:19.2", "38:19.3", "38:19.3", "38:19.3", "38:19.4", "38:19.4", "38:19.4", "38:19.5", "38:19.5", "38:19.5", "38:19.6", "38:19.6", "38:19.6", "38:19.7", "38:19.7", "38:19.7", "38:19.8", "38:19.8", "38:19.8", "38:19.9", "38:19.9", "38:19.9", "38:20.0", "38:20.0", "38:20.0", "38:20.1", "38:20.1", "38:20.1", "38:20.2", "38:20.2", "38:20.2", "38:20.3", "38:20.3", "38:20.3", "38:20.4", "38:20.4", "38:20.4", "38:20.5", "38:20.5", "38:20.5", "38:20.6", "38:20.6", "38:20.6", "38:20.7", "38:20.7", "38:20.7", "38:20.8", "38:20.8", "38:20.8", "38:20.9", "38:20.9", "38:20.9", "38:21.0", "38:21.0", "38:21.0", "38:21.1", "38:21.1", "38:21.1", "38:21.2", "38:21.2", "38:21.2", "38:21.3", "38:21.3", "38:21.3", "38:21.4", "38:21.4", "38:21.4", "38:21.5", "38:21.5", "38:21.5", "38:21.6", "38:21.6", "38:21.6", "38:21.7", "38:21.7", "38:21.7", "38:21.8", "38:21.8", "38:21.8", "38:21.9", "38:21.9", "38:21.9", "38:22.0", "38:22.0", "38:22.0", "38:22.1", "38:22.1", "38:22.1", "38:22.2", "38:22.2", "38:22.2", "38:22.3", "38:22.3", "38:22.3", "38:22.4", "38:22.4", "38:22.4", "38:22.5", "38:22.5", "38:22.5", "38:22.6", "38:22.6", "38:22.6", "38:22.7", "38:22.7", "38:22.7", "38:22.8", "38:22.8", "38:22.8", "38:22.9", "38:22.9", "38:22.9", "38:23.0", "38:23.0", "38:23.0", "38:23.1", "38:23.1", "38:23.1", "38:23.2", "38:23.2", "38:23.2", "38:23.3", "38:23.3", "38:23.3", "38:23.4", "38:23.4", "38:23.4", "38:23.5", "38:23.5", "38:23.5", "38:23.6", "38:23.6", "38:23.6", "38:23.7", "38:23.7", "38:23.7", "38:23.8", "38:23.8", "38:23.8", "38:23.9", "38:23.9", "38:23.9", "38:24.0", "38:24.0", "38:24.0", "38:24.1", "38:24.1", "38:24.1", "38:24.2", "38:24.2", "38:24.2", "38:24.3", "38:24.3", "38:24.3", "38:24.4", "38:24.4", "38:24.4", "38:24.5", "38:24.5", "38:24.5", "38:24.6", "38:24.6", "38:24.6", "38:24.7", "38:24.7", "38:24.7", "38:24.8", "38:24.8", "38:24.8", "38:24.9", "38:24.9", "38:24.9", "38:25.0", "38:25.0", "38:25.0", "38:25.1", "38:25.1", "38:25.1", "38:25.2", "38:25.2", "38:25.2", "38:25.3", "38:25.3", "38:25.3", "38:25.4", "38:25.4", "38:25.4", "38:25.5", "38:25.5", "38:25.5", "38:25.6", "38:25.6", "38:25.6", "38:25.7", "38:25.7", "38:25.7", "38:25.8", "38:25.8", "38:25.8", "38:25.9", "38:25.9", "38:25.9", "38:26.0", "38:26.0", "38:26.0", "38:26.1", "38:26.1", "38:26.1", "38:26.2", "38:26.2", "38:26.2", "38:26.3", "38:26.3", "38:26.3", "38:26.4", "38:26.4", "38:26.4", "38:26.5", "38:26.5", "38:26.5", "38:26.6", "38:26.6", "38:26.6", "38:26.7", "38:26.7", "38:26.7", "38:26.8", "38:26.8", "38:26.8", "38:26.9", "38:26.9", "38:26.9", "38:27.0", "38:27.0", "38:27.0", "38:27.1", "38:27.1", "38:27.1", "38:27.2", "38:27.2", "38:27.2", "38:27.3", "38:27.3", "38:27.3", "38:27.4", "38:27.4", "38:27.4", "38:27.5", "38:27.5", "38:27.5", "38:27.6", "38:27.6", "38:27.6", "38:27.7", "38:27.7", "38:27.7", "38:27.8", "38:27.8", "38:27.8", "38:27.9", "38:27.9", "38:27.9", "38:28.0", "38:28.0", "38:28.0", "38:28.1", "38:28.1", "38:28.1", "38:28.2", "38:28.2", "38:28.2", "38:28.3", "38:28.3", "38:28.3", "38:28.4", "38:28.4", "38:28.4", "38:28.5", "38:28.5", "38:28.5", "38:28.6", "38:28.6", "38:28.6", "38:28.7", "38:28.7", "38:28.7", "38:28.8", "38:28.8", "38:28.8", "38:28.9", "38:28.9", "38:28.9", "38:29.0", "38:29.0", "38:29.0", "38:29.1", "38:29.1", "38:29.1", "38:29.2", "38:29.2", "38:29.2", "38:29.3", "38:29.3", "38:29.3", "38:29.4", "38:29.4", "38:29.4", "38:29.5", "38:29.5", "38:29.5", "38:29.6", "38:29.6", "38:29.6", "38:29.7", "38:29.7", "38:29.7", "38:29.8", "38:29.8", "38:29.8", "38:29.9", "38:29.9", "38:29.9", "38:30.0", "38:30.0", "38:30.0", "38:30.1", "38:30.1", "38:30.1", "38:30.2", "38:30.2", "38:30.2", "38:30.3", "38:30.3", "38:30.3", "38:30.4", "38:30.4", "38:30.4", "38:30.5", "38:30.5", "38:30.5", "38:30.6", "38:30.6", "38:30.6", "38:30.7", "38:30.7", "38:30.7", "38:30.8", "38:30.8", "38:30.8", "38:30.9", "38:30.9", "38:30.9", "38:31.0", "38:31.0", "38:31.0", "38:31.1", "38:31.1", "38:31.1", "38:31.2", "38:31.2", "38:31.2", "38:31.3", "38:31.3", "38:31.3", "38:31.4", "38:31.4", "38:31.4", "38:31.5", "38:31.5", "38:31.5", "38:31.6", "38:31.6", "38:31.6", "38:31.7", "38:31.7", "38:31.7", "38:31.8", "38:31.8", "38:31.8", "38:31.9", "38:31.9", "38:31.9", "38:32.0", "38:32.0", "38:32.0", "38:32.1", "38:32.1", "38:32.1", "38:32.2", "38:32.2", "38:32.2", "38:32.3", "38:32.3", "38:32.3", "38:32.4", "38:32.4", "38:32.4", "38:32.5", "38:32.5", "38:32.5", "38:32.6", "38:32.6", "38:32.6", "38:32.7", "38:32.7", "38:32.7", "38:32.8", "38:32.8", "38:32.8", "38:32.9", "38:32.9", "38:32.9", "38:33.0", "38:33.0", "38:33.0", "38:33.1", "38:33.1", "38:33.1", "38:33.2", "38:33.2", "38:33.2", "38:33.3", "38:33.3", "38:33.3", "38:33.4", "38:33.4", "38:33.4", "38:33.5", "38:33.5", "38:33.5", "38:33.6", "38:33.6", "38:33.6", "38:33.7", "38:33.7", "38:33.7", "38:33.8", "38:33.8", "38:33.8", "38:33.9", "38:33.9", "38:33.9", "38:34.0", "38:34.0", "38:34.0", "38:34.1", "38:34.1", "38:34.1", "38:34.2", "38:34.2", "38:34.2", "38:34.3", "38:34.3", "38:34.3", "38:34.4", "38:34.4", "38:34.4", "38:34.5", "38:34.5", "38:34.5", "38:34.6", "38:34.6", "38:34.6", "38:34.7", "38:34.7", "38:34.7", "38:34.8", "38:34.8", "38:34.8", "38:34.9", "38:34.9", "38:34.9", "38:35.0", "38:35.0", "38:35.0", "38:35.1", "38:35.1", "38:35.1", "38:35.2", "38:35.2", "38:35.2", "38:35.3", "38:35.3", "38:35.3", "38:35.4", "38:35.4", "38:35.4", "38:35.5", "38:35.5", "38:35.5", "38:35.6", "38:35.6", "38:35.6", "38:35.7", "38:35.7", "38:35.7", "38:35.8", "38:35.8", "38:35.8", "38:35.9", "38:35.9", "38:35.9", "38:36.0", "38:36.0", "38:36.0", "38:36.1", "38:36.1", "38:36.1", "38:36.2", "38:36.2", "38:36.2", "38:36.3", "38:36.3", "38:36.3", "38:36.4", "38:36.4", "38:36.4", "38:36.5", "38:36.5", "38:36.5", "38:36.6", "38:36.6", "38:36.6", "38:36.7", "38:36.7", "38:36.7", "38:36.8", "38:36.8", "38:36.8", "38:36.9", "38:36.9", "38:36.9", "38:37.0", "38:37.0", "38:37.0", "38:37.1", "38:37.1", "38:37.1", "38:37.2", "38:37.2", "38:37.2", "38:37.3", "38:37.3", "38:37.3", "38:37.4", "38:37.4", "38:37.4", "38:37.5", "38:37.5", "38:37.5", "38:37.6", "38:37.6", "38:37.6", "38:37.7", "38:37.7", "38:37.7", "38:37.8", "38:37.8", "38:37.8", "38:37.9", "38:37.9", "38:37.9", "38:38.0", "38:38.0", "38:38.0", "38:38.1", "38:38.1", "38:38.1", "38:38.2", "38:38.2", "38:38.2", "38:38.3", "38:38.3", "38:38.3", "38:38.4", "38:38.4", "38:38.4", "38:38.5", "38:38.5", "38:38.5", "38:38.6", "38:38.6", "38:38.6", "38:38.7", "38:38.7", "38:38.7", "38:38.8", "38:38.8", "38:38.8", "38:38.9", "38:38.9", "38:38.9", "38:39.0", "38:39.0", "38:39.0", "38:39.1", "38:39.1", "38:39.1", "38:39.2", "38:39.2", "38:39.2", "38:39.3", "38:39.3", "38:39.3", "38:39.4", "38:39.4", "38:39.4", "38:39.5", "38:39.5", "38:39.5", "38:39.6", "38:39.6", "38:39.6", "38:39.7", "38:39.7", "38:39.7", "38:39.8", "38:39.8", "38:39.8", "38:39.9", "38:39.9", "38:39.9", "38:40.0", "38:40.0", "38:40.0", "38:40.1", "38:40.1", "38:40.1", "38:40.2", "38:40.2", "38:40.2", "38:40.3", "38:40.3", "38:40.3", "38:40.4", "38:40.4", "38:40.4", "38:40.5", "38:40.5", "38:40.5", "38:40.6", "38:40.6", "38:40.6", "38:40.7", "38:40.7", "38:40.7", "38:40.8", "38:40.8", "38:40.8", "38:40.9", "38:40.9", "38:40.9", "38:41.0", "38:41.0", "38:41.0", "38:41.1", "38:41.1", "38:41.1", "38:41.2", "38:41.2", "38:41.2", "38:41.3", "38:41.3", "38:41.3", "38:41.4", "38:41.4", "38:41.4", "38:41.5", "38:41.5", "38:41.5", "38:41.6", "38:41.6", "38:41.6", "38:41.7", "38:41.7", "38:41.7", "38:41.8", "38:41.8", "38:41.8", "38:41.9", "38:41.9", "38:41.9", "38:42.0", "38:42.0", "38:42.0", "38:42.1", "38:42.1", "38:42.1", "38:42.2", "38:42.2", "38:42.2", "38:42.3", "38:42.3", "38:42.3", "38:42.4", "38:42.4", "38:42.4", "38:42.5", "38:42.5", "38:42.5", "38:42.6", "38:42.6", "38:42.6", "38:42.7", "38:42.7", "38:42.7", "38:42.8", "38:42.8", "38:42.8", "38:42.9", "38:42.9", "38:42.9", "38:43.0", "38:43.0", "38:43.0", "38:43.1", "38:43.1", "38:43.1", "38:43.2", "38:43.2", "38:43.2", "38:43.3", "38:43.3", "38:43.3", "38:43.4", "38:43.4", "38:43.4", "38:43.5", "38:43.5", "38:43.5", "38:43.6", "38:43.6", "38:43.6", "38:43.7", "38:43.7", "38:43.7", "38:43.8", "38:43.8", "38:43.8", "38:43.9", "38:43.9", "38:43.9", "38:44.0", "38:44.0", "38:44.0", "38:44.1", "38:44.1", "38:44.1", "38:44.2", "38:44.2", "38:44.2", "38:44.3", "38:44.3", "38:44.3", "38:44.4", "38:44.4", "38:44.4", "38:44.5", "38:44.5", "38:44.5", "38:44.6", "38:44.6", "38:44.6", "38:44.7", "38:44.7", "38:44.7", "38:44.8", "38:44.8", "38:44.8", "38:44.9", "38:44.9", "38:44.9", "38:45.0", "38:45.0", "38:45.0", "38:45.1", "38:45.1", "38:45.1", "38:45.2", "38:45.2", "38:45.2", "38:45.3", "38:45.3", "38:45.3", "38:45.4", "38:45.4", "38:45.4", "38:45.5", "38:45.5", "38:45.5", "38:45.6", "38:45.6", "38:45.6", "38:45.7", "38:45.7", "38:45.7", "38:45.8", 
